vi "BuildArenaSQLString.vi"(11 "BattleLog":T1) -> (3 "SQL INSERT request":string)   [LabVIEW 2020, in "StashRoyale.lvclass"]
uses:
  StashRoyale.lvclass
  ctl_BattleLog.ctl
  ctl_Team.ctl
  ctl_CardTeam.ctl
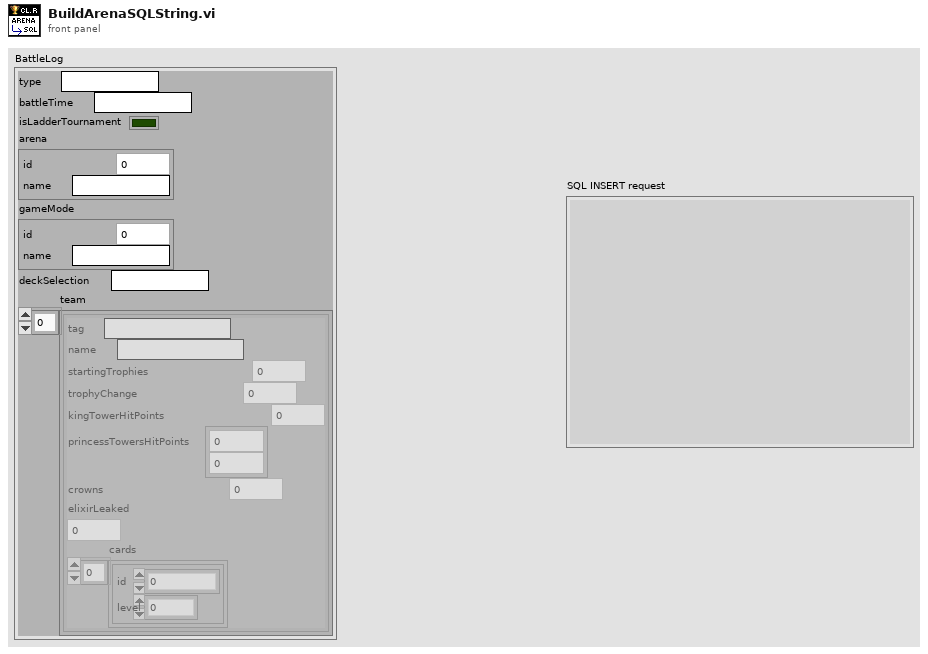
[diagram p1: front panel]
types:
  T1 = typedef "StashRoyale.lvclass/ctl_BattleLog.ctl" = cluster{"type":string, "battleTime":string, "isLadderTournament":bool, "arena":cluster{"id":u32, "name":string}, "gameMode":cluster{"id":u32, "name":string}, "deckSelection":string, "team":T2[]}
  T2 = typedef "ctl_Team.ctl" = cluster{"tag":string, "name":string, "startingTrophies":u16, "trophyChange":i16, "kingTowerHitPoints":u16, "princessTowersHitPoints":u16[], "crowns":u16, "elixirLeaked":sgl, "cards":T3[]}
  T3 = typedef "StashRoyale.lvclass/ctl_CardTeam.ctl" = cluster{"id":u32, "level":u8}
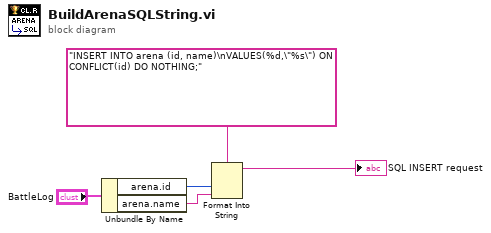
[diagram p0: block diagram]
diagram:
  n1 = Unbundle By Name("BattleLog") -> ("arena.id"=w3:u32, "arena.name"=w1:string)
  n2 = Format Into String(format string="INSERT INTO arena (id, name)\nVALUES(%d,\"%s\") ON CONFLICT(id) DO NOTHING;", w3, w1) -> (resulting string=→"SQL INSERT request":string)  [unwired: 2 in, 1 out]
